vi "Disc Eject System.vi"(11 "Disc Eject":bool) -> ()   [LabVIEW 2018]
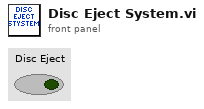
[diagram p1: front panel]
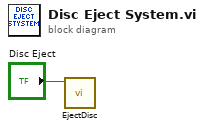
[diagram p0: block diagram]
diagram:
  n1 = call "EjectDisc.vi"("Disc Eject"="Disc Eject") -> ()  [unwired: 11 in]
